vi "Update Configuration from Target.vi"(8 "error in (no error)":errorcluster, 11 "Configuration Cluster":refnum<vi>) -> (0 "error out":errorcluster)   [LabVIEW 2017]
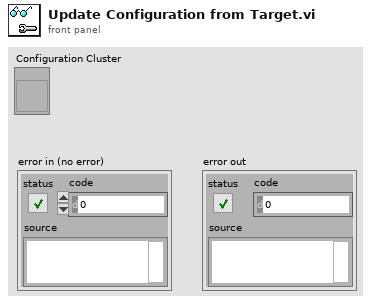
[diagram p1: front panel]
types:
  T1 = cluster{"Center Frequency":u32, "Sample Rate (Bandwidth)":u32, "Tuner AGC Mode":bool, "AGC Mode":bool, "Manual Gain":u16, "Number of Averages":u32, "Frequency Correction":i32}
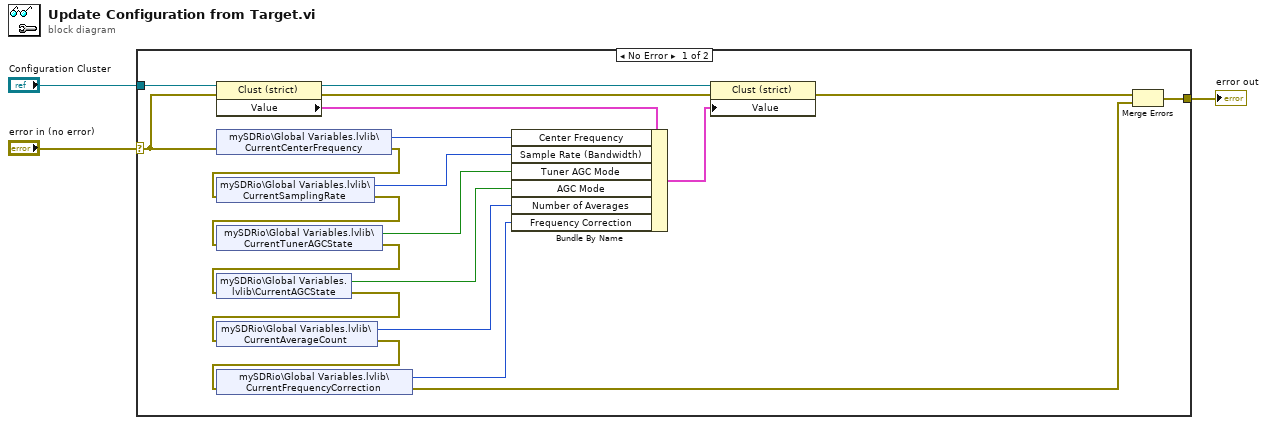
[diagram p0: block diagram]
diagram:
  n1 = case shown="No Error" "error in (no error)" {
    selector: "error in (no error)" -> [w17 w24]
    tunnel: [w18 w24] -> w2
    tunnel: "Configuration Cluster" -> [w16 _]
    frame No Error {
      n2 = property on="Property Node" class="Clust (strict)"(reference=w16, error in=w17) -> (reference out=w15:refnum<vi>, error out=w23:errorcluster, "Value"=w22:T1)
      n3 = shared-variable "mySDRio\\Global Variables.lvlib\\CurrentCenterFrequency"(error in=w17) -> (w21:u32, error out=w9:errorcluster)
      n4 = shared-variable "mySDRio\\Global Variables.lvlib\\CurrentSamplingRate"(error in=w9) -> (w14:u32, error out=w8:errorcluster)
      n5 = shared-variable "mySDRio\\Global Variables.lvlib\\CurrentTunerAGCState"(error in=w8) -> (w13:bool, error out=w7:errorcluster)
      n6 = shared-variable "mySDRio\\Global Variables.lvlib\\CurrentAGCState"(error in=w7) -> (w12:bool, error out=w6:errorcluster)
      n7 = shared-variable "mySDRio\\Global Variables.lvlib\\CurrentAverageCount"(error in=w6) -> (w11:u32, error out=w5:errorcluster)
      n8 = shared-variable "mySDRio\\Global Variables.lvlib\\CurrentFrequencyCorrection"(error in=w5) -> (w10:i32, error out=w4:errorcluster)
      n9 = Bundle By Name(cluster=w22, "Center Frequency"=w21, "Sample Rate (Bandwidth)"=w14, "Tuner AGC Mode"=w13, "AGC Mode"=w12, "Number of Averages"=w11, "Frequency Correction"=w10) -> (w20:T1)
      n10 = property on="Property Node" class="Clust (strict)"(reference=w15, error in=w23, "Value"=w20) -> (error out=w19:errorcluster)  [unwired: 1 out]
      n11 = Merge Errors(w19, w4) -> (w18:errorcluster)
    }
    frame Error {
    }
  }
  "error out" <- w2
